vi "StripEmtyLines.vi"(0 "Path":path) -> ()   [LabVIEW 2013]
uses:
  <vilib>/regexp/Match Regular Expression.xnode
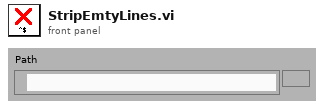
[diagram p1: front panel]
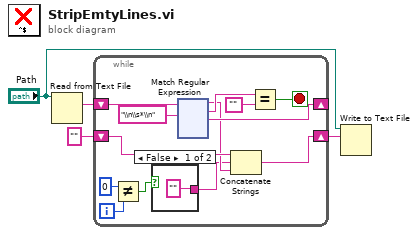
[diagram p0: block diagram]
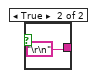
[diagram p2: hidden frame]
diagram:
  n1 = Read from Text File(file (use dialog)="Path") -> (text=w4:string)  [unwired: 3 in, 3 out]
  n2 = while {
    shift-right: [w13] -> _
    shift-left: w4 -> [w14]
    shift-right: [w10] -> w2
    shift-left: "" ("before match") -> [w11]
    i -> [w6]
    stop <- w15 stop-if-true
    n3 = Not Equal?(x=0, y=w6) -> (x != y?=w7:bool)
    n4 = case shown="False" w7 {
      tunnel: ["" ("before match") "\r\n" ("before match")] -> w8
      frame False {
      }
      frame True {
      }
    }
    n5 = xnode "Match Regular Expression"("input string"=w14, "regular expression"="\\n\\s*\\n") -> ("before match"=w9:string, "whole match"=w17:string, "after match"=w13:string)  [unwired: 4 in, 2 out]
    n6 = Concatenate Strings(w11, w8, w9) -> (w10:string)
    n7 = Equal?(x=w17, y="") -> (x = y?=w15:bool)
  }
  n8 = Write to Text File(file (use dialog)="Path", text=w2) -> ()  [unwired: 2 in, 3 out]
